vi "4461 - Stop Tasks.vi"(8 "error in (no error)":errorcluster, 11 "Lockin":refnum<class "Instrument.Lockin.lvclass">) -> (0 "error out":errorcluster, 3 "Lockin out":refnum<class "Instrument.Lockin.lvclass">)   [LabVIEW 2016, in "Instrument.Lockin.lvclass"]
uses:
  Instrument.Lockin.lvclass
  Instrument.Lockin.lvclass/Instrument.Lockin.ctl
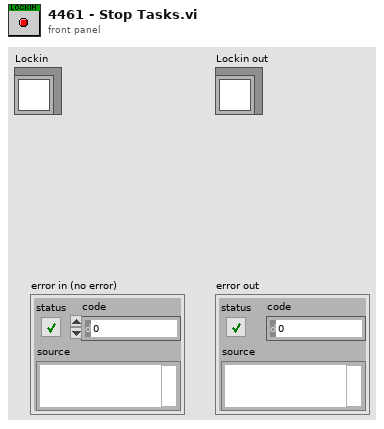
[diagram p1: front panel]
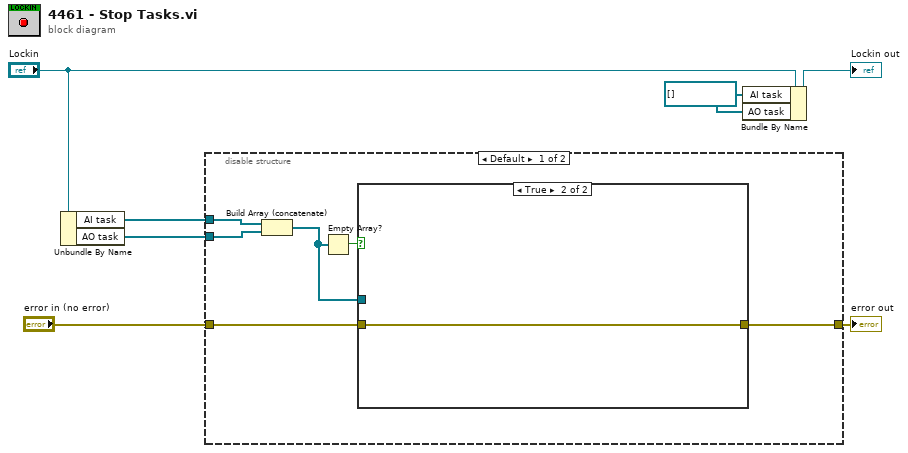
[diagram p0: block diagram]
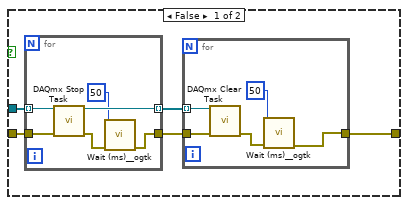
[diagram p2: hidden frame]
diagram:
  w2 = refnum<k21>[] [] ("AI task")
  n1 = Unbundle By Name("Lockin") -> ("AI task"=w4:refnum<k21>[], "AO task"=w5:refnum<k21>[])
  n2 = disable-structure shown="Default" {
    disable-tunnel: "error in (no error)" -> [w13 _]
    disable-tunnel: [w9 _] -> w6
    disable-tunnel: w5 -> [w11 _]
    disable-tunnel: w4 -> [w12 _]
    frame condition #0 (active) {
      n3 = Build Array (concatenate)(w12, w11) -> (w10:refnum<k21>[])
      n4 = Empty Array?(array=w10) -> (empty?=w8:bool)
      n5 = case shown="True" w8 {
        tunnel: w13 -> [w18 w30]
        tunnel: w10 -> [w15 _]
        tunnel: [w14 w30] -> w9
        frame False {
          n6 = for {
            tunnel: w15 -> [w29] mode=indexing
            tunnel: [w28] -> w17 mode=indexing
            tunnel: w18 -> [w27]
            tunnel: [w25] -> w16
            n7 = call <vilib>:"DAQmx Stop Task.vi"("task/channels in"=w29, "error in"=w27) -> ("task out"=w28:refnum<k21>, "error out"=w26:errorcluster)  [unwired: 12 in]
            n8 = call <userlib>:"Wait (ms)__ogtk.vi"("error in (no error)"=w26, "milliseconds to wait"=u32 50) -> ("error out"=w25:errorcluster)  [unwired: 8 in, 1 out]
          }
          n9 = for {
            tunnel: w17 -> [w23] mode=indexing
            tunnel: w16 -> [w22]
            tunnel: [w19] -> w14
            n10 = call <vilib>:"DAQmx Clear Task.vi"("task in"=w23, "error in"=w22) -> ("error out"=w20:errorcluster)  [unwired: 13 in]
            n11 = call <userlib>:"Wait (ms)__ogtk.vi"("error in (no error)"=w20, "milliseconds to wait"=u32 50) -> ("error out"=w19:errorcluster)  [unwired: 8 in, 1 out]
          }
        }
        frame True {
        }
      }
    }
    frame condition #1 {
    }
  }
  "error out" <- w6
  n12 = Bundle By Name(cluster="Lockin", "AI task"=w2, "AO task"=w2) -> (→"Lockin out":refnum<class "Instrument.Lockin.lvclass">)
